vi "BufferSizeTracepoint.vi"(10 "Buffer Size":i32, 11 "Qbus":refnum<class "Qbus.lvclass">) -> ()   [LabVIEW 2017]
uses:
  <vilib>/addons/Qbus/Qbus.lvclass
  <vilib>/addons/TraceLogger/TraceLogger.lvlib
  <vilib>/addons/InsightCM/Devices/Shared/Common/DataAccumulator/DataAccumulator.lvlib
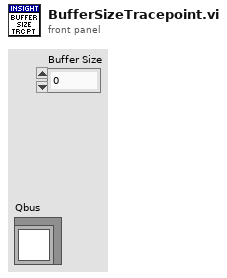
[diagram p1: front panel]
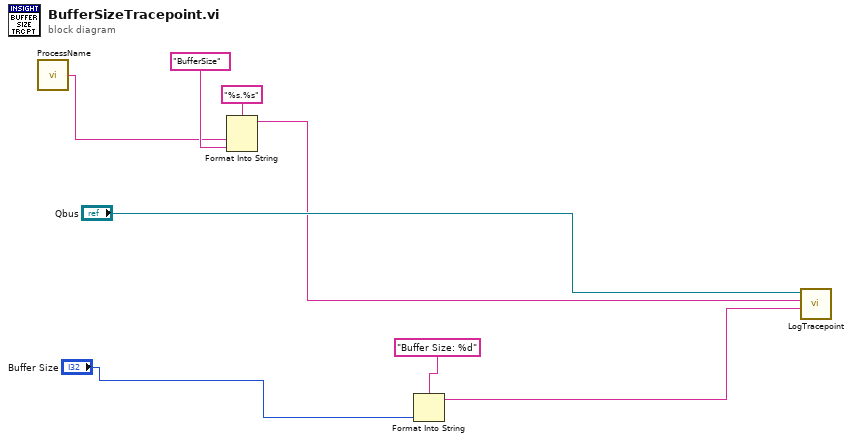
[diagram p0: block diagram]
diagram:
  n1 = call <vilib>:"ProcessName.vi"() -> ("process name"=w1:string)  [unwired: 5 in]
  n2 = Format Into String(format string="%s.%s", w1, "BufferSize" ("tracepoint")) -> (resulting string=w4:string)  [unwired: 2 in, 1 out]
  n3 = Format Into String(format string="Buffer Size: %d", "Buffer Size") -> (resulting string=w3:string)  [unwired: 2 in, 1 out]
  n4 = call <vilib>:"LogTracepoint.vi"("log string"=w3, "tracepoint"=w4, "qbus in"="Qbus") -> ()  [unwired: 7 in, 2 out]
